vi "运维调试_采配水V2.vi"() -> ()   [LabVIEW 2016, in "PLC.lvlib"]
uses:
  PLC.lvlib
  <vilib>/Plasmionique/MB Master/MB_Master/MB_Master.lvclass
  <vilib>/Utility/miscctls.llb/LVPointTypeDef.ctl
  <vilib>/Plasmionique/MB Master/MB_Master_Serial/MB_Master_Serial.lvclass
  C:/Program Files (x86)/National Instruments/LabVIEW 2016/vi.lib/Plasmionique/MB Master/MB_Master/MB_Master.lvclass
  <vilib>/Instr/_visa.llb/VISA Configure Serial Port (Instr).vi
  <vilib>/NI/Modbus Library/API/Wrapper/Create TCP Slave.vi
  <vilib>/NI/Modbus Library/API/slave/Modbus Slave.lvclass
  <vilib>/Plasmionique/MB Master/MB Master.lvlib
  <vilib>/NI/Modbus Library/API/Wrapper/API Main.lvlib
panel:
  out "Registers":u16[](array[numeric])
  out "R118":i16 caption="多参数沉淀时间"
  in  "看门狗启用":bool
  out "R117":i16 caption="看门狗设置值"
  out "R33":i16 caption="看门狗计时器"
  in  "下载模式":bool
  in  "R116":i16(ring) caption="储水水体选择" items=["自来水", "采水泵"]
  out "当前启动泵号":u16(ring) items=["1号水样泵", "2号水样泵"]
  out "R113":i16 caption="储水时间设定"
  out "R25":i16
  in  "V14NC":bool
  out "R24":i16
  in  "V14NO":bool
  out "X2":bool caption="X1"
  out "采配水版本号":string
  out "R23":i16 caption="清洗频次计数"
  out "R112":i16 caption="清洗频次设定"
  out "R22":i16
  in  "V13NC":bool
  out "R111":i16 caption="排液时间"
  out "通讯故障":bool
  out "R21":i16
  in  "V13NO":bool
  out "R20":i16
  in  "M1-2":bool
  in  "潜水泵工作模式":u16(ring) items=["泵1单泵单管路", "泵2单泵单管路", "潜水泵双泵双管路", "自吸泵双泵双管路"]
  out "X11":bool caption="废液报警"
  out "X10":bool caption="自来水检测"
  out "X9":bool caption="泵2过载报警"
  out "X8":bool caption="泵1过载报警"
  out "X7":bool caption="断电检测"
  out "X6":bool caption="开门检测"
  out "X5":bool caption="烟雾检测"
  out "X4":bool caption="漏水检测"
  out "X3":bool caption="进样检测"
  out "X1":bool
  out "X0":bool caption="采样池液位开关"
  out "R109":i16 caption="配水时间"
  out "集成报警信息":string
  out "R108":i16 caption="自来水报警"
  out "R107":i16 caption="采水池液位报警设置"
  out "R106":i16 caption="进样超时设置"
  out "R105":i16 caption="二级清洗时间"
  out "R104":i16 caption="一级清洗时间"
  out "R103":i16 caption="外部管路清洗时间"
  out "R102":i16 caption="静置沉淀时间"
  out "R101":i16 caption="内部管路润洗时间"
  out "R100":i16 caption="外部管路润洗时间"
  out "R2":i16
  out "R1":i16
  out "多列列表框":i32(listbox)
  out "R19":i16
  in  "V6":bool
  out "R18":i16
  in  "V5":bool
  out "R17":i16
  in  "V4":bool
  out "R16":i16
  in  "V3":bool
  out "R15":i16
  in  "V2":bool
  out "R14":i16
  in  "M2":bool
  out "R13":i16
  in  "V1":bool
  out "R12":i16
  in  "M1-1":bool
  in  "返回":bool
  in  "参数设置":bool
  in  "单步启动":bool
  in  "启动":bool
  in  "停止":bool
  # "看门狗设置"
  # "S"
  # "S"
  # "S"
  # "S"
  # "次"
  # "次"
  # "S"
  # "S"
  # "S"
  # "S"
  # "S"
  # "S"
  # "S"
  # "S"
  # "S"
  # "S"
  # "S"
  # "单步计时："
  # "s"
  # "流程计时："
  # "s"
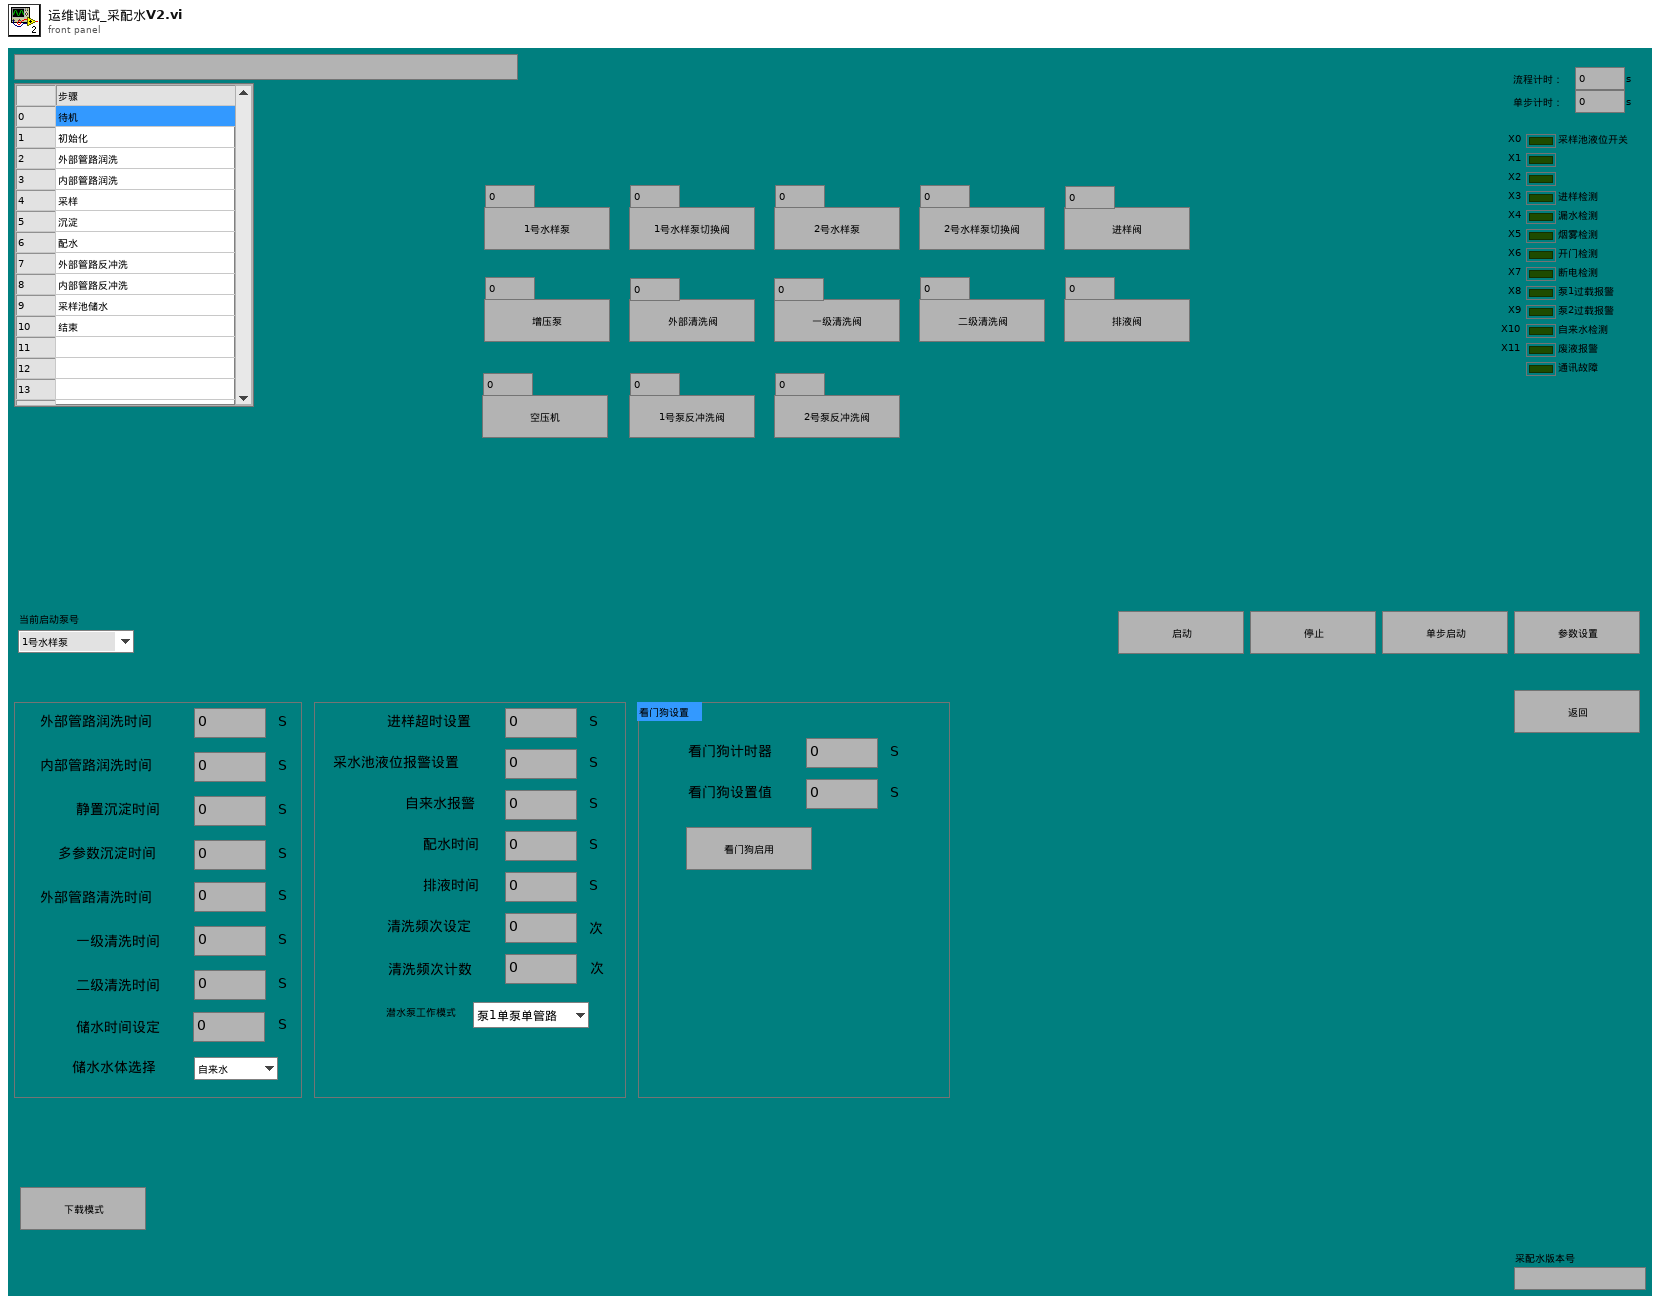
[diagram p1: front panel]
types:
  T1 = typedef "LVPointTypeDef.ctl" = cluster{"Horizontal":i16, "Vertical":i16}
  T2 = cluster{"命令":string, "数据":cluster{"starting address":u16, "holding register value":u16}}
  T3 = cluster{"时间标识":timestamp, "设备":string, "日志信息":string}
  T4 = cluster{"R0":i16, "R1":i16, "R2":i16, "R3":i16, "R4":i16, "R5":i16, "R6":i16, "R7":i16, "R8":i16, "R9":i16, "R10":i16, "R11":i16, "R12":i16, "R13":i16, "R14":i16, "R15":i16, "R16":i16, "R17":i16, "R18":i16, "R19":i16, "R20":i16, "R21":i16, "R22":i16, "R23":i16, "R24":i16, "R25":i16, "R26":i16, "R27":i16, "R28":i16, "R29":i16, "R30":i16, "R31":i16, "R32":i16, "R33":i16, "R34":i16}
  T5 = cluster{"R100":i16, "R101":i16, "R102":i16, "R103":i16, "R104":i16, "R105":i16, "R106":i16, "R107":i16, "R108":i16, "R109":i16, "R110":i16, "R111":i16, "R112":i16, "R113":i16, "R114":i16, "R115":i16, "R116":i16, "R117":i16, "R118":i16, "R119":i16}
  T6 = cluster{"seconds since 1Jan1904":timestamp, "table输入":string, string, "table输入":string}
  T7 = cluster{"时间标识":timestamp, "设备":string, "日志信息":string, "流程参数":string}
  T8 = cluster{"命令":string, cluster{"starting address":u16, "holding register value":u16}}
  T9 = cluster{"命令":string, "数据":cluster{"starting address":u16, "holding register values":u16[]}}
  T10 = cluster{"命令":string, "data":cluster{"starting address":u16, "coil values":bool[]}}
  T11 = cluster{"测试模式":enum16{"正常测试", "集成干预"}, "参数启用":cluster{"氨氮":bool, "总磷总氮":bool, "CODMn":bool, "CODcr":bool, "多参数":bool, "超标留样":bool}}
  T12 = enum32{"Bad", "Idle", "Run top level", "Running"}
  T13 = cluster{"baud rate (bps)":u32, "stop bits":u16, "parity":u16, "flow control":u16, "timeout":u32, "retries":i32}
  T14 = cluster{"starting address":u16, "holding register values":u16[]}
  T15 = cluster{"starting address":u16, "holding register value":u16}
  T16 = cluster{"starting address":u16, "coil values":bool[]}
  T17 = cluster{"Registers[0]":u16, "Registers[1]":u16, "Registers[2]":u16, "Registers[3]":u16, "Registers[4]":u16, "Registers[5]":u16, "Registers[6]":u16, "Registers[7]":u16, "Registers[8]":u16, "Registers[9]":u16, "Registers[10]":u16, "Registers[11]":u16, "Registers[12]":u16, "Registers[13]":u16, "Registers[14]":u16, "Registers[15]":u16, "Registers[16]":u16, "Registers[17]":u16, "Registers[18]":u16, "Registers[19]":u16, "Registers[20]":u16, "Registers[21]":u16, "Registers[22]":u16, "Registers[23]":u16, "Registers[24]":u16, "Registers[25]":u16, "Registers[26]":u16, "Registers[27]":u16, "Registers[28]":u16, "Registers[29]":u16, "Registers[30]":u16, "Registers[31]":u16, "Registers[32]":u16, "Registers[33]":u16, "Registers[34]":u16}
  T18 = cluster{"数组 2[0]":sgl, "数组 2[1]":sgl, "数组 2[2]":sgl, "数组 2[3]":sgl, "数组 2[4]":sgl}
  T19 = cluster{"Registers[0]":u16, "Registers[1]":u16, "Registers[2]":u16, "Registers[3]":u16, "Registers[4]":u16, "Registers[5]":u16}
  T20 = cluster{"Registers[0]":u16, "Registers[1]":u16, "Registers[2]":u16, "Registers[3]":u16, "Registers[4]":u16, "Registers[5]":u16, "Registers[6]":u16, "Registers[7]":u16, "Registers[8]":u16, "Registers[9]":u16, "Registers[10]":u16, "Registers[11]":u16, "Registers[12]":u16, "Registers[13]":u16, "Registers[14]":u16, "Registers[15]":u16, "Registers[16]":u16, "Registers[17]":u16, "Registers[18]":u16, "Registers[19]":u16}
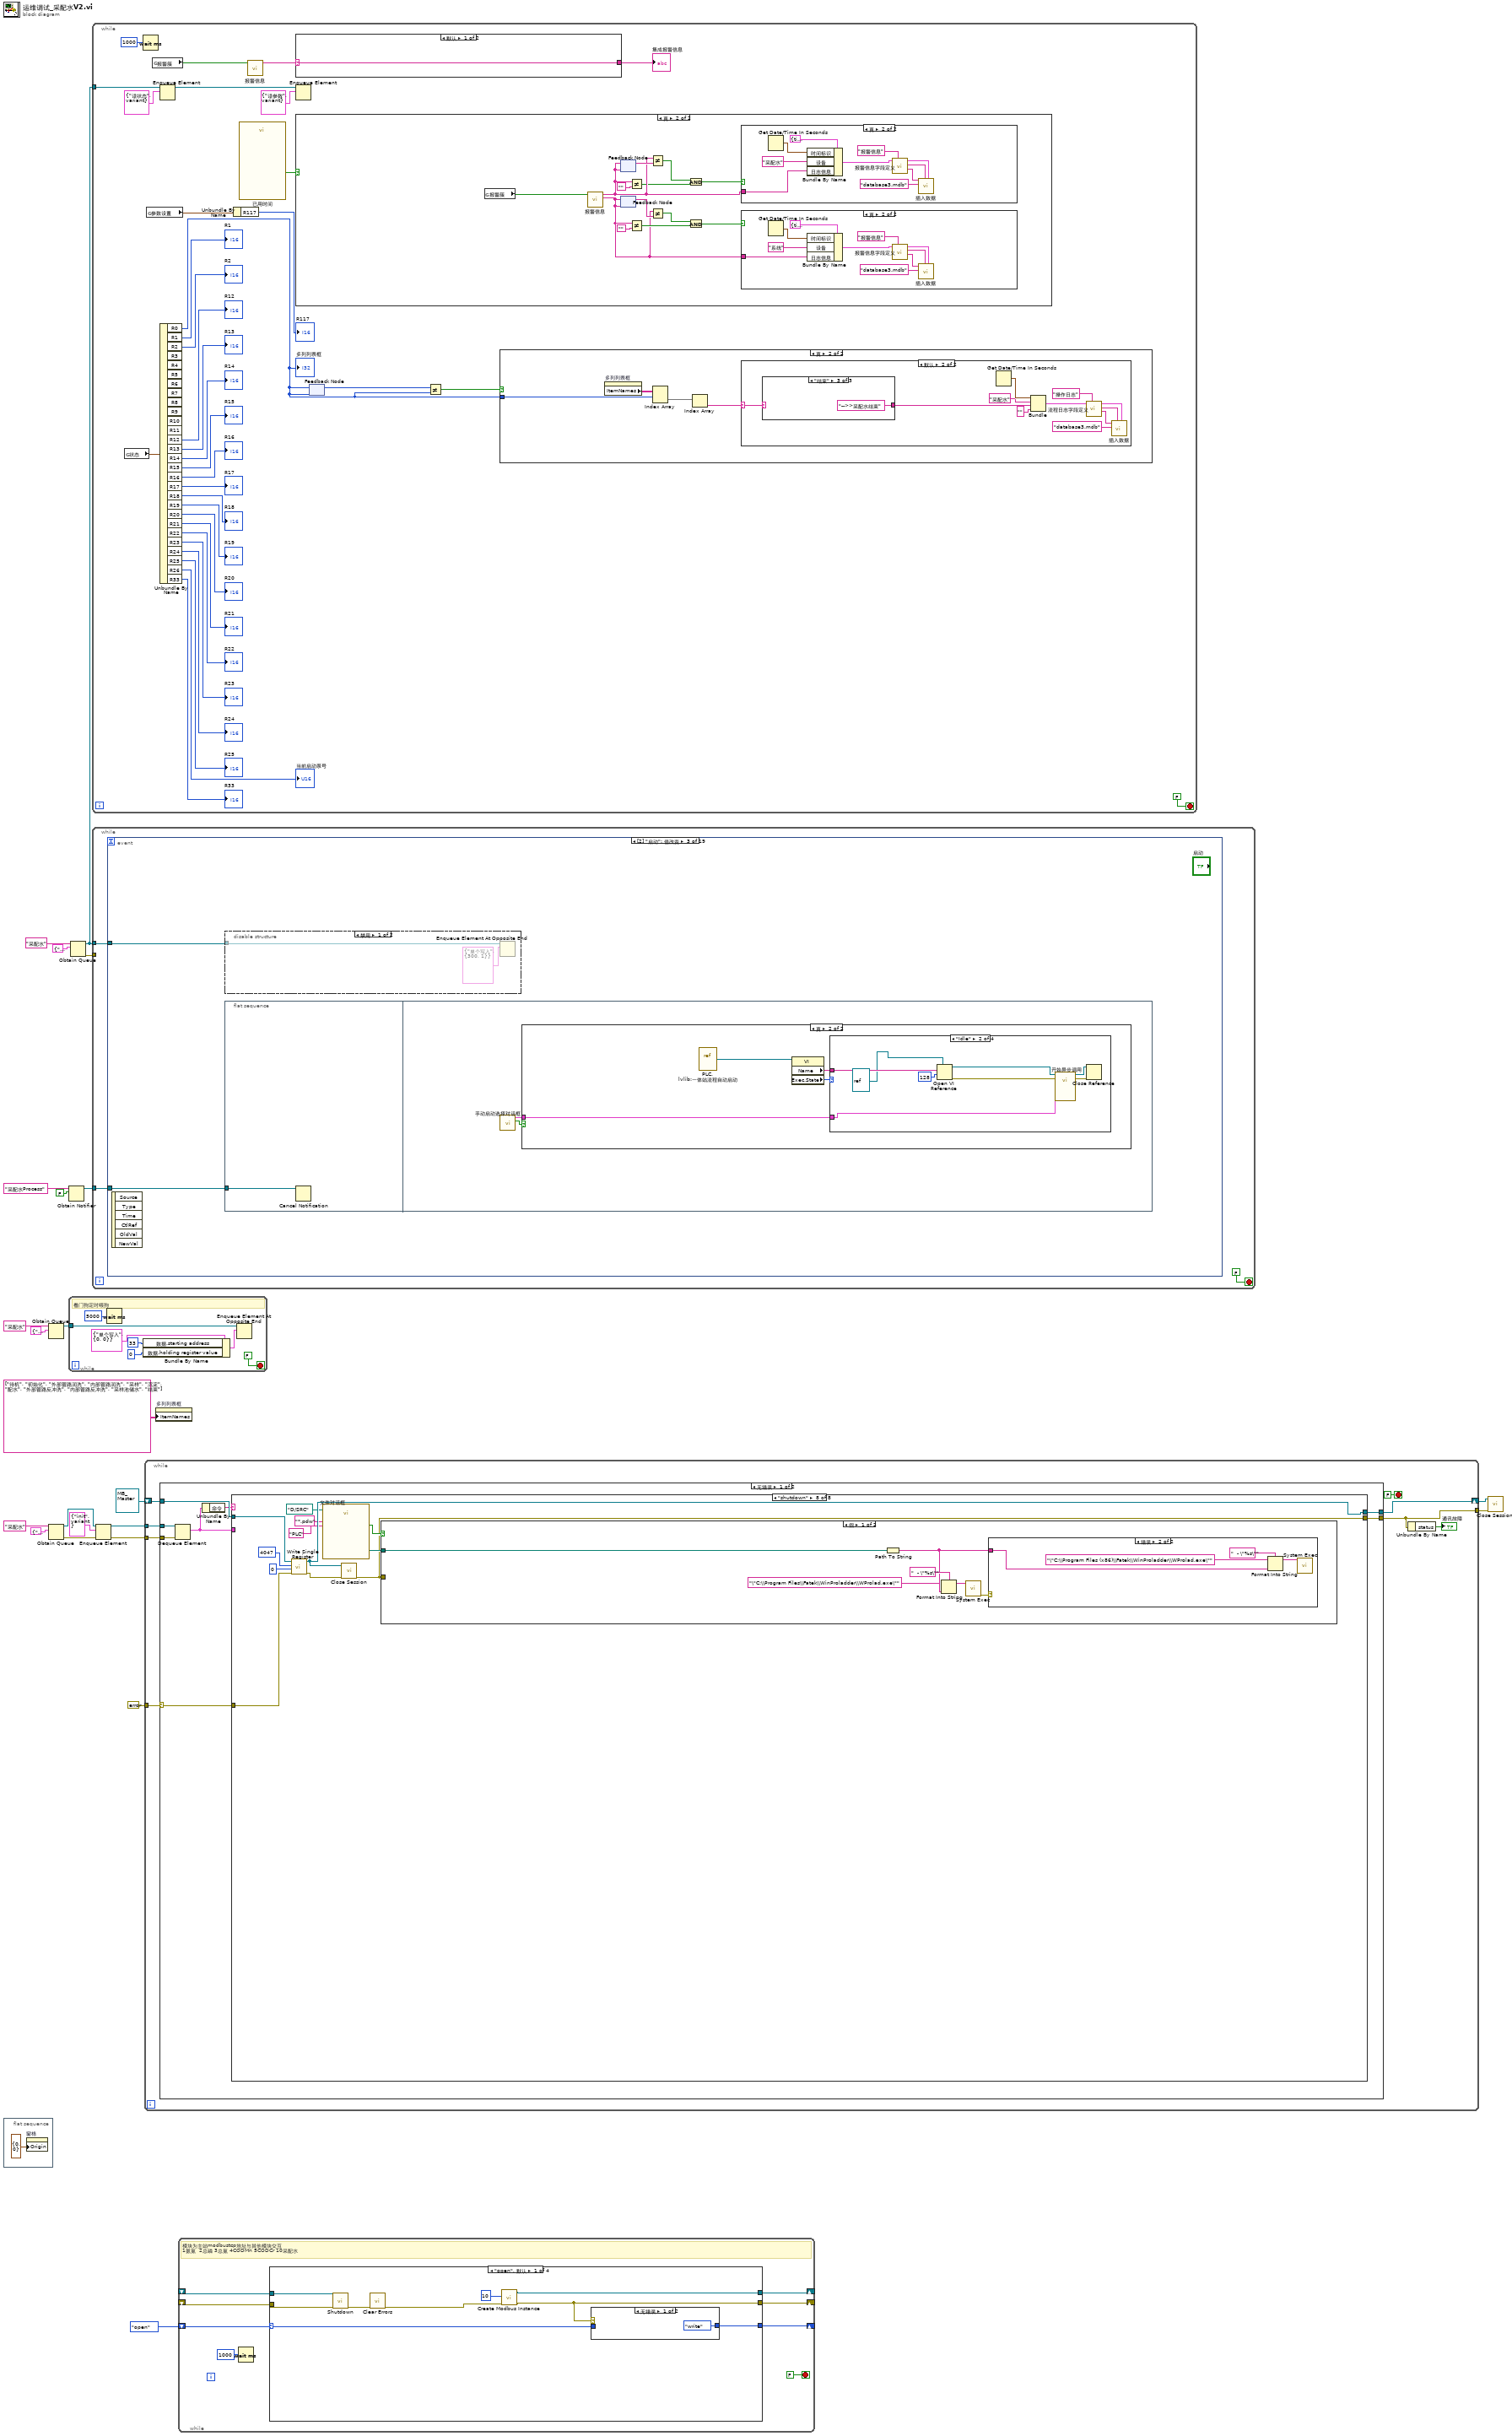
[diagram p0: block diagram]
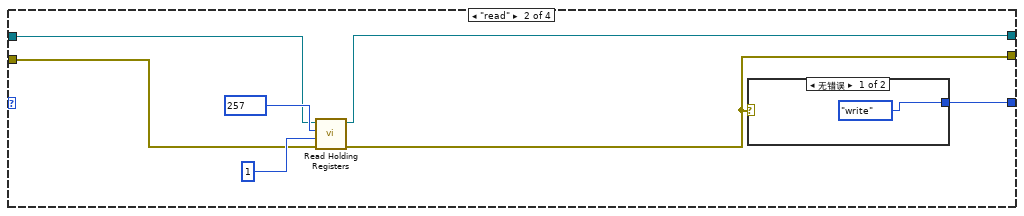
[diagram p3: hidden frame]
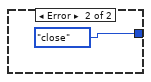
[diagram p4: hidden frame]
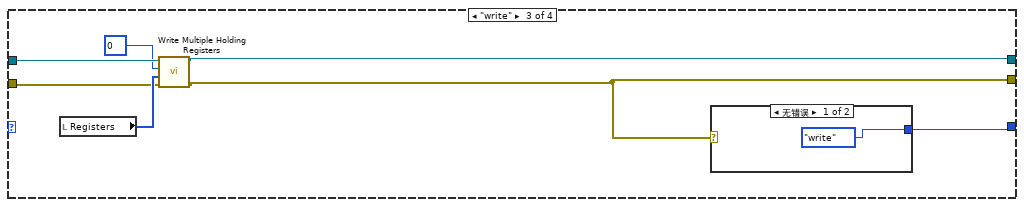
[diagram p5: hidden frame]
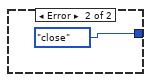
[diagram p6: hidden frame]
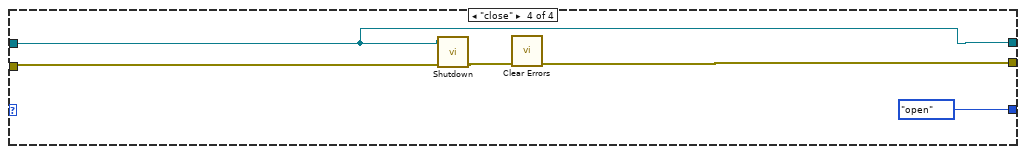
[diagram p7: hidden frame]
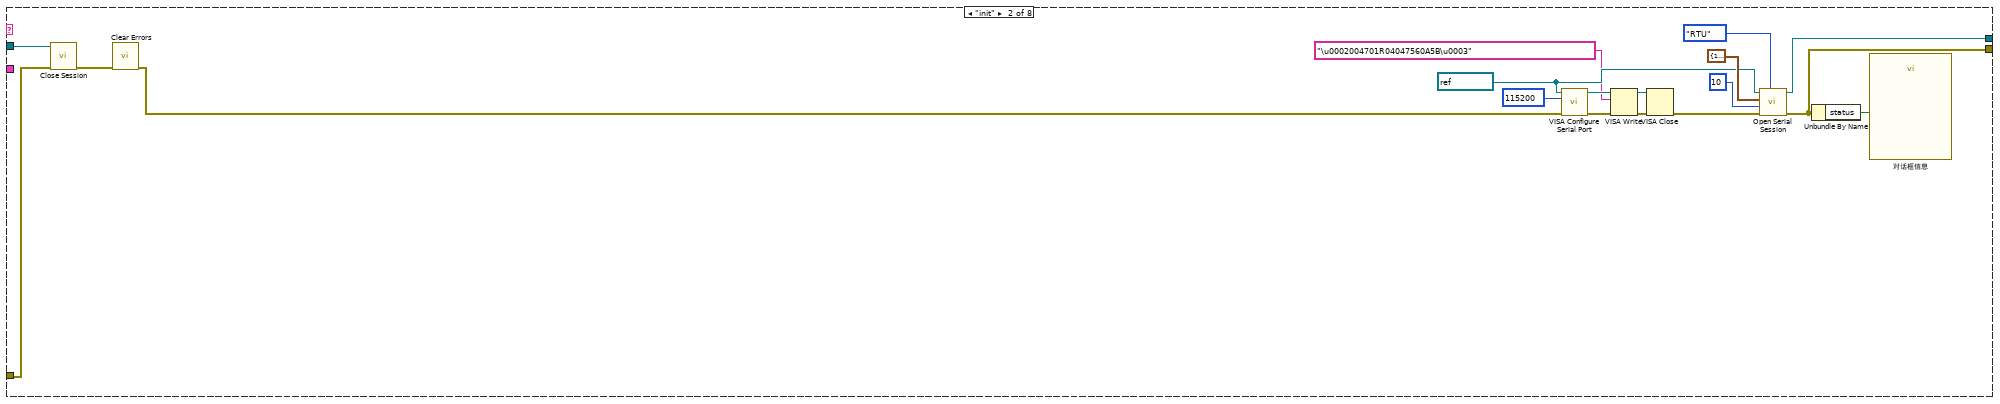
[diagram p9: hidden frame]
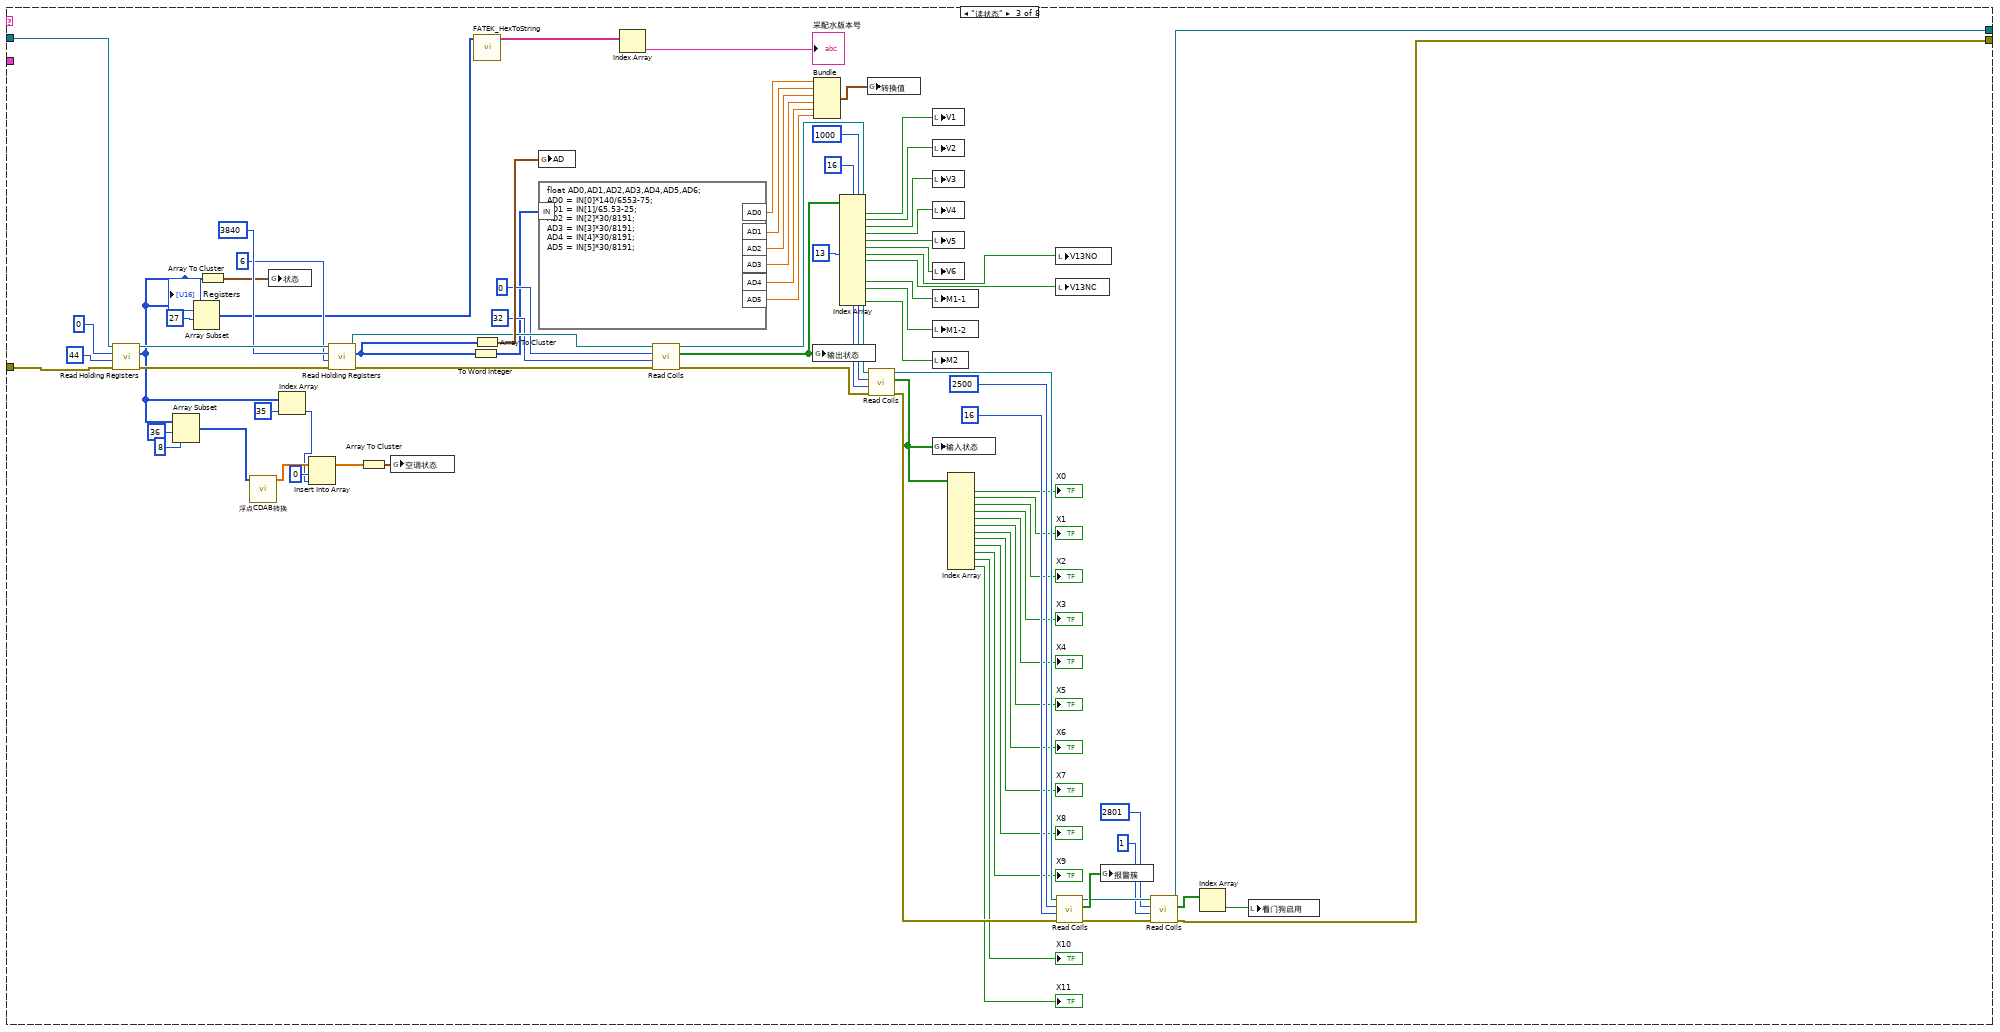
[diagram p10: hidden frame]
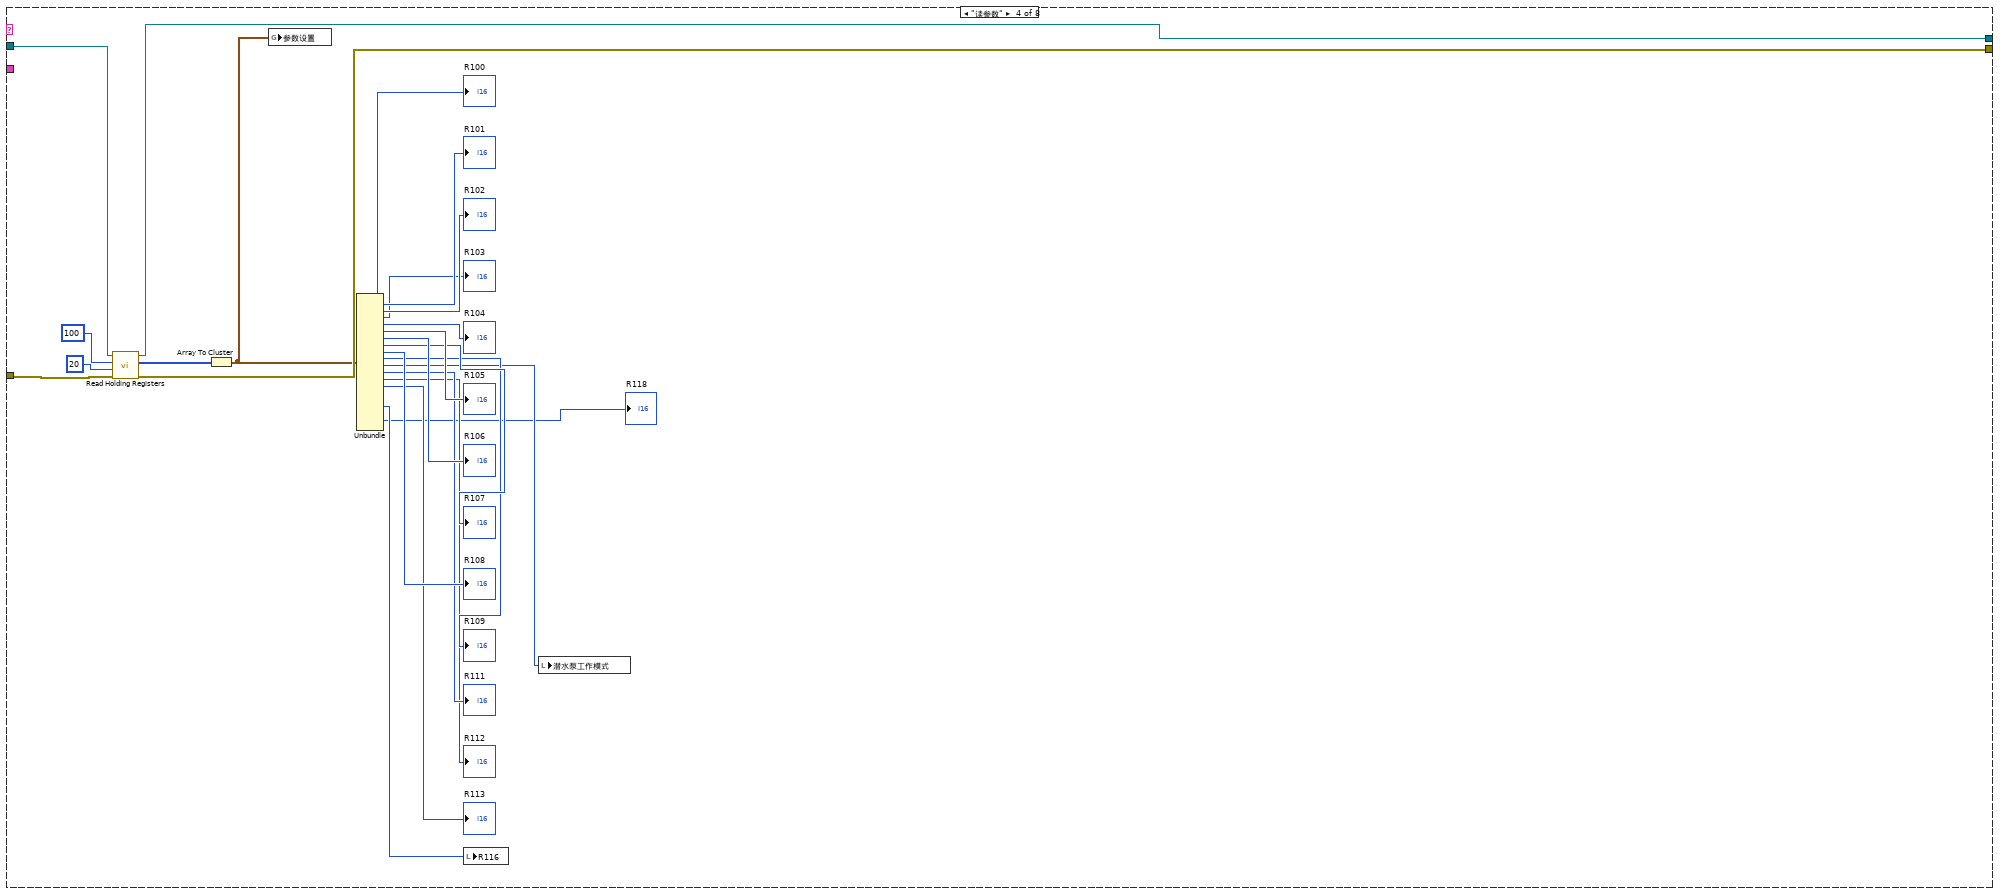
[diagram p11: hidden frame]
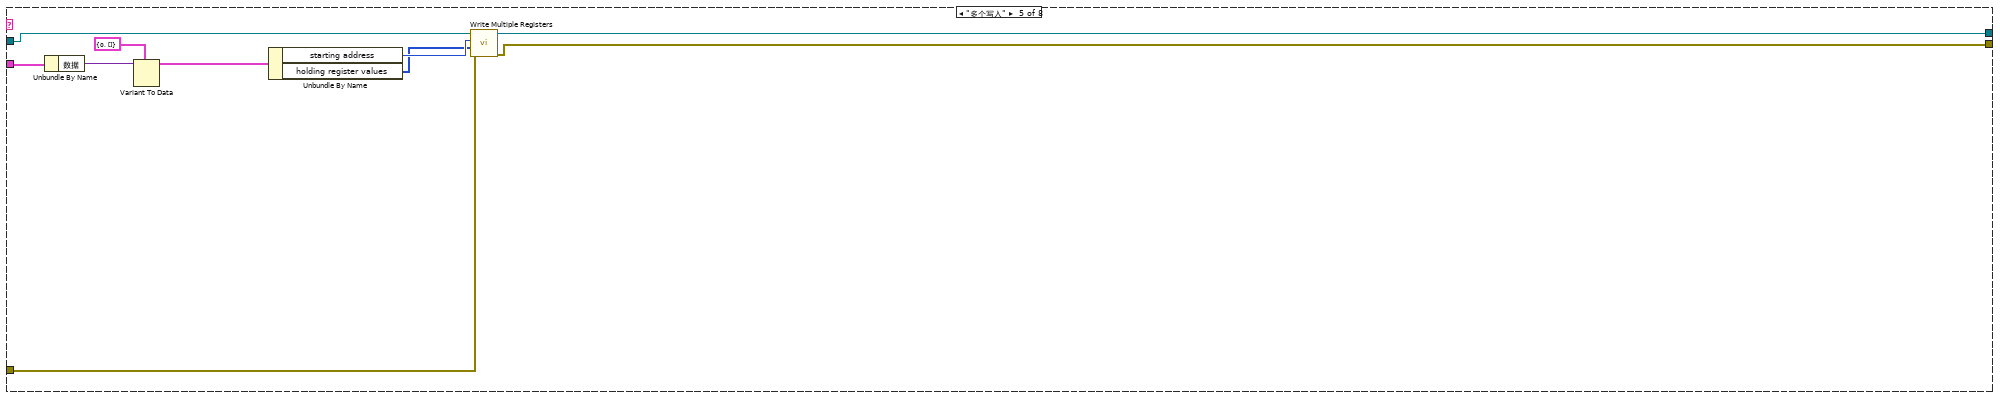
[diagram p12: hidden frame]
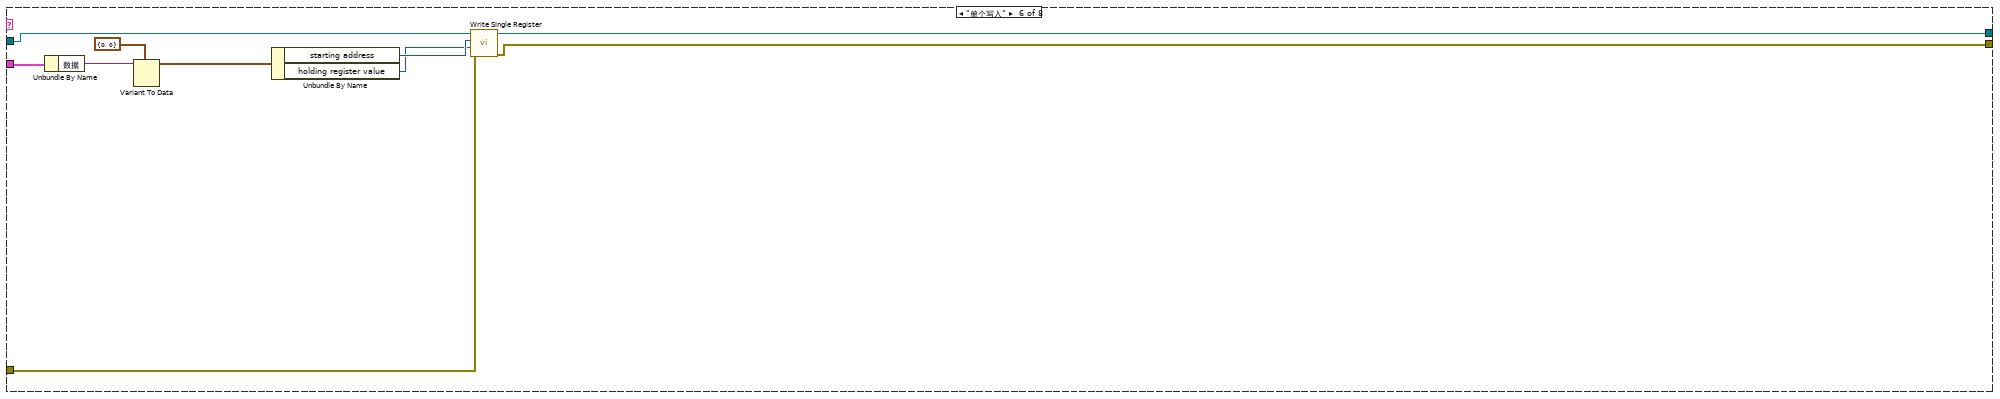
[diagram p13: hidden frame]
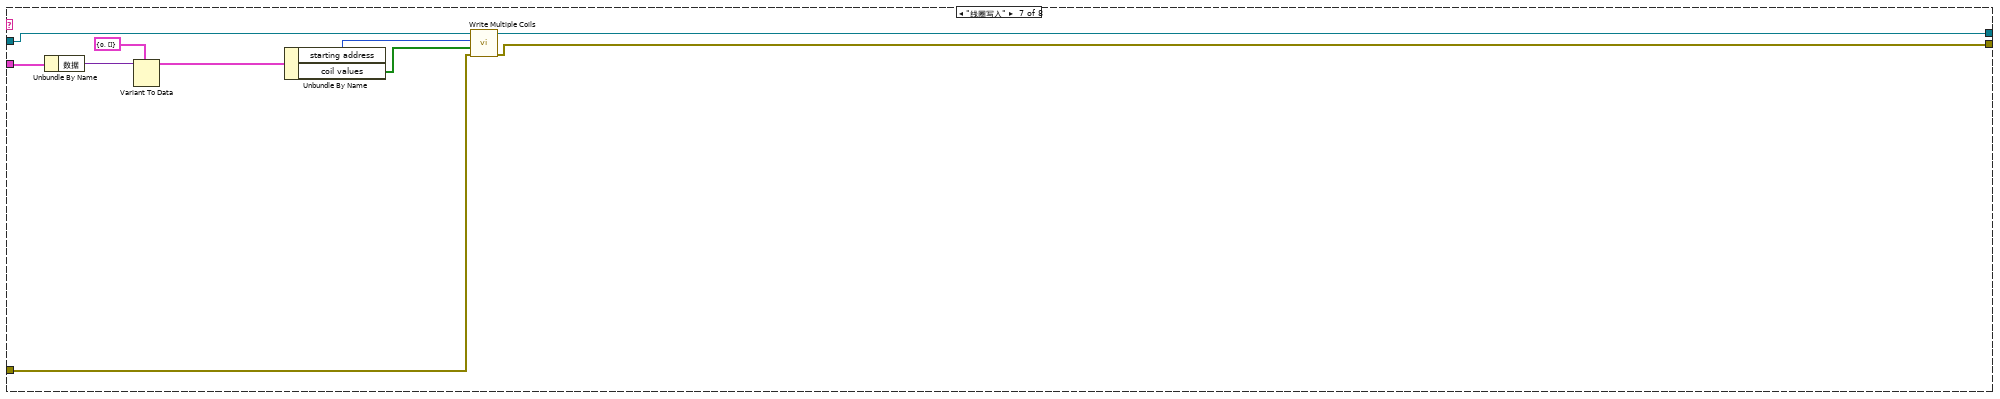
[diagram p14: hidden frame]
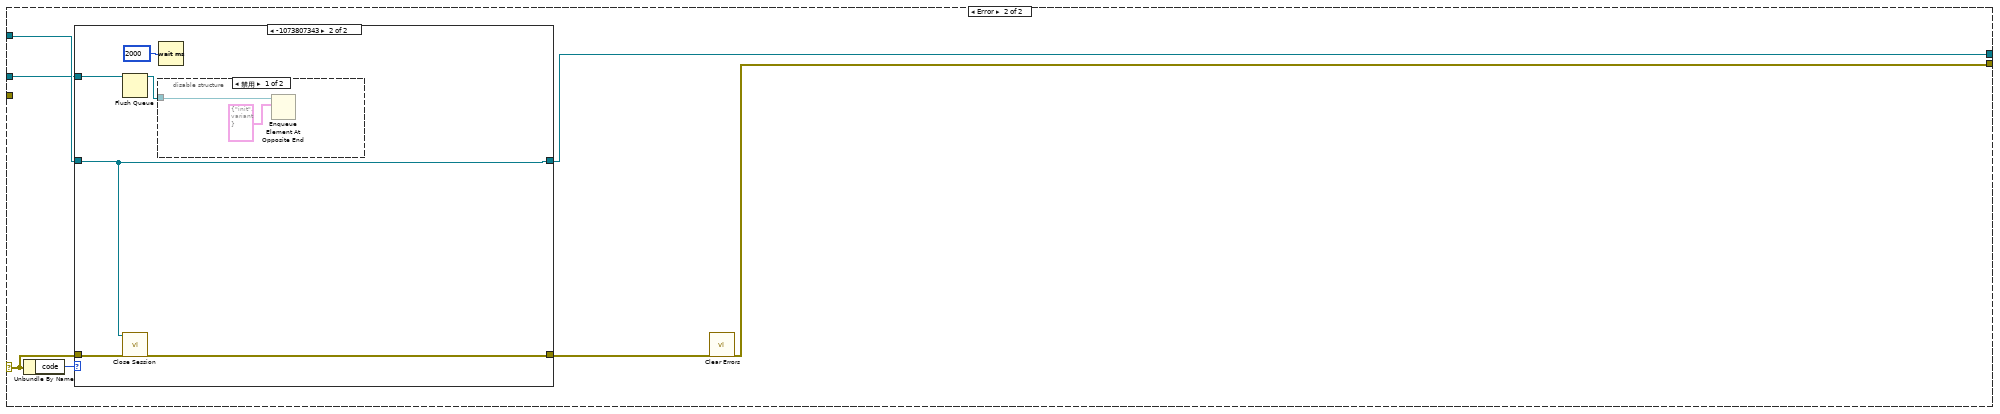
[diagram p17: hidden frame]
diagram:
  n1 = flat-sequence {
    frame #0 {
      n2 = property on="窗格" class="Pane"("Origin"=T1 {"Horizontal"=0, "Vertical"=0} ("原点")) -> ()  [unwired: 2 in, 2 out]
    }
  }
  n3 = Obtain Queue(name (unnamed)="采配水" ("名称（未命名）"), element data type=cluster{"命令":string, "数据":variant} {"命令"="", "数据"=variant}) -> (queue out=w2:refnum<queue>)  [unwired: 3 in, 2 out]
  n4 = Obtain Queue(name (unnamed)="采配水" ("名称（未命名）"), element data type=cluster{"命令":string, "数据":variant} {"命令"="", "数据"=variant}) -> (queue out=w13:refnum<queue>, error out=w12:errorcluster)  [unwired: 3 in, 1 out]
  n5 = Obtain Notifier(name (unnamed)="采配水Process" ("名称（未命名）"), notification data type=FALSE) -> (notifier out=w16:refnum<notifier>)  [unwired: 2 in, 2 out]
  n6 = while {
    tunnel: w2 -> [w27]
    stop <- FALSE stop-if-true
    # "看门狗定时喂狗"
    n7 = Wait (ms)(milliseconds to wait=u32 5000 ("等待时间（毫秒）")) -> ()  [unwired: 1 out]
    n8 = Bundle By Name(cluster=T2 {"命令"="单个写入", "数据"={"starting address"=0, "holding register value"=0}} ("元素"), "数据.starting address"=u16 33, "数据.holding register value"=u16 0) -> (w28:T2)
    n9 = Enqueue Element At Opposite End(queue=w27, element=w28) -> ()  [unwired: 2 in, 3 out]
  }
  n10 = Obtain Queue(name (unnamed)="采配水" ("名称（未命名）"), element data type=cluster{"命令":string, "数据":variant} {"命令"="", "数据"=variant}) -> (queue out=w20:refnum<queue>, error out=w21:errorcluster)  [unwired: 3 in, 1 out]
  n11 = while {
    tunnel: w20 -> [w64]
    stop <- FALSE stop-if-true
    n12 = global read "采配水全局变量.vi" "状态"() -> (w62:T4)
    n13 = Wait (ms)(milliseconds to wait=u32 1000 ("等待时间（毫秒）")) -> ()  [unwired: 1 out]
    n14 = global read "采配水全局变量.vi" "参数设置"() -> (w33:T5)
    n15 = global read "采配水全局变量.vi" "报警簇"() -> (w50:bool[])
    n16 = Enqueue Element(queue=w64, element=cluster{"命令":string, "数据":variant} {"命令"="读状态", "数据"=variant} ("元素")) -> (queue out=w45:refnum<queue>)  [unwired: 2 in, 2 out]
    n17 = Unbundle By Name(w62) -> ("R0"=w43:i16, "R1"=→"R1":i16, "R2"=→"R2":i16, "R12"=→"R12":i16, "R13"=→"R13":i16, "R14"=→"R14":i16, "R15"=→"R15":i16, "R16"=→"R16":i16, "R17"=→"R17":i16, "R18"=→"R18":i16, "R19"=→"R19":i16, "R20"=→"R20":i16, "R21"=→"R21":i16, "R22"=→"R22":i16, "R23"=→"R23":i16, "R24"=→"R24":i16, "R25"=→"R25":i16, "R26"=→"当前启动泵号":i16, "R33"=→"R33":i16)  [unwired: 9 out]
    "多列列表框" <- w43
    n18 = Unbundle By Name(w33) -> ("R117"=→"R117":i16)
    n19 = call "已用时间"() -> ("Time has Elapsed"=w48:bool)  [unwired: 12 in, 7 out]
    n20 = call "报警信息.vi"("报警簇"=w50) -> ("采配水报警信息"=w42:string)  [unwired: 9 in, 1 out]
    n21 = case shown="默认" w42 {
      selector: w42 -> [w99 _]
      tunnel: [w99 w100] -> w49
      frame Default {
      }
      frame "" {
        n22 = global read "采配水全局变量.vi" "运行状态显示"() -> (w100:string)
      }
    }
    "集成报警信息" <- w49
    n23 = Enqueue Element(queue=w45, element=cluster{"命令":string, "数据":variant} {"命令"="读参数", "数据"=variant} ("元素")) -> ()  [unwired: 2 in, 3 out]
    n24 = case shown="真" w48 {
      frame False {
      }
      frame True {
        n25 = global read "采配水全局变量.vi" "报警簇"() -> (w78:bool[])
        n26 = call "报警信息.vi"("报警簇"=w78) -> ("系统报警信息"=w67:string, "采配水报警信息"=w74:string)  [unwired: 9 in]
        n27 = feedback #1(w74) -> (w77:string)
        n28 = feedback-in #1(w74) -> ()
        n29 = feedback #2(w67) -> (w68:string)
        n30 = feedback-in #2(w67) -> ()
        n31 = Not Equal?(x=w74, y="") -> (x != y?=w72:bool)
        n32 = Not Equal?(x=w67, y="") -> (x != y?=w71:bool)
        n33 = Not Equal?(x=w74, y=w77) -> (x != y?=w76:bool)
        n34 = Not Equal?(x=w67, y=w68) -> (x != y?=w69:bool)
        n35 = And(x=w76, y=w72) -> (x .and. y?=w75:bool)
        n36 = And(x=w69, y=w71) -> (x .and. y?=w66:bool)
        n37 = case shown="真" w75 {
          tunnel: w74 -> [_ w89]
          frame False {
          }
          frame True {
            n38 = Get Date/Time In Seconds() -> (seconds since 1Jan1904=w91:timestamp)
            n39 = Bundle By Name(cluster=T3 {"时间标识"=timestamp(0 s since 1904-01-01), "设备"="", "日志信息"=""} ("data in"), "时间标识"=w91, "设备"="采配水", "日志信息"=w89) -> (w92:T3)
            n40 = call "报警信息字段定义.vi"("table输入"="报警信息", "data in"=w92) -> ("table输出"=w96:string, "columns"=w97:string[], "data out"=w98:T3)  [unwired: 7 in]
            n41 = call "插入数据.vi"("data"=w98, "columns"=w97, "database"="database3.mdb", "table"=w96) -> ()  [unwired: 7 in, 1 out]
          }
        }
        n42 = case shown="真" w66 {
          tunnel: w67 -> [_ w79]
          frame False {
          }
          frame True {
            n43 = Get Date/Time In Seconds() -> (seconds since 1Jan1904=w81:timestamp)
            n44 = Bundle By Name(cluster=T3 {"时间标识"=timestamp(0 s since 1904-01-01), "设备"="", "日志信息"=""} ("data in"), "时间标识"=w81, "设备"="系统", "日志信息"=w79) -> (w82:T3)
            n45 = call "报警信息字段定义.vi"("table输入"="报警信息", "data in"=w82) -> ("table输出"=w86:string, "columns"=w87:string[], "data out"=w88:T3)  [unwired: 7 in]
            n46 = call "插入数据.vi"("data"=w88, "columns"=w87, "database"="database3.mdb", "table"=w86) -> ()  [unwired: 7 in, 1 out]
          }
        }
      }
    }
    n47 = feedback-in #3(w43) -> ()
    n48 = feedback #3(w43) -> (w44:i16)
    n49 = Not Equal?(x=w44, y=w43) -> (x != y?=w51:bool)
    n50 = case shown="真" w51 {
      tunnel: w43 -> [_ w103]
      frame False {
      }
      frame True {
        n51 = property on="多列列表框" class="MCListbox (严格)"() -> ("ItemNames"=w104:string[][])  [unwired: 2 in, 2 out]
        n52 = Index Array(array=w104, index (row)=w103) -> (element=w102:string[])  [unwired: 1 in]
        n53 = Index Array(array=w102) -> (element=w101:string)  [unwired: 1 in]
        n54 = case shown="默认" w101 {
          selector: w101 -> [_ w106]
          frame "待机" {
          }
          frame Default {
            n55 = case shown="\"结束\"" w106 {
              selector: w106 -> [w116 _ _]
              tunnel: [w116 "-->>采配水初始化" "-->>采配水结束"] -> w105
              frame Default {
              }
              frame "初始化" {
              }
              frame "结束" {
              }
            }
            n56 = Get Date/Time In Seconds() -> (seconds since 1Jan1904=w110:timestamp)
            n57 = Bundle("seconds since 1Jan1904"=w110, "table输入"="采配水", w105, "table输入"="") -> (w108:T6)  [unwired: 1 in]
            n58 = call "流程日志字段定义.vi"("table输入"="操作日志", "data in"=w108) -> ("table输出"=w113:string, "columns"=w114:string[], "data out"=w115:T7)  [unwired: 7 in]
            n59 = call "插入数据.vi"("data"=w115, "columns"=w114, "database"="database3.mdb", "table"=w113) -> ()  [unwired: 7 in, 1 out]
          }
        }
      }
    }
  }
  n60 = while {
    tunnel: w20 -> [w120]
    tunnel: w21 -> [_]
    tunnel: w16 -> [w119]
    stop <- FALSE stop-if-true
    n61 = event shown="[2] \"启动\": 值改变" {
      selector: _ -> [_ _ _ _ _ _ _ _ _ _ _ _ _ _ _ _ _ _ _]
      dyn-events: _ -> [_ _ _ _ _ _ _ _ _ _ _ _ _ _ _ _ _ _ _]
      timeout: _ -> [_ _ _ _ _ _ _ _ _ _ _ _ _ _ _ _ _ _ _]
      tunnel: w120 -> [_ w124 w127 w149 w168 w173 w179 w190 _ _ _ _ w218 w220 w225 w230 w235 w240 w245]
      tunnel: w119 -> [_ w123 w126 _ _ _ _ _ _ _ _ _ _ _ _ _ _ _ _]
      event Timeout {
        n62 = event-data() -> ()  [unwired: 1 in, 3 out]
      }
      event "停止": Value Change {
        n63 = event-data() -> ()  [unwired: 1 in, 6 out]
        n64 = Send Notification(notification=TRUE ("通知"), notifier=w123) -> ()  [unwired: 1 in, 2 out]
        n65 = Enqueue Element At Opposite End(queue=w124, element=T8 {"命令"="单个写入", {"starting address"=300, "holding register value"=2}} ("元素")) -> ()  [unwired: 2 in, 3 out]
      }
      event "启动": Value Change {
        n66 = event-data() -> ()  [unwired: 1 in, 6 out]
        n67 = disable-structure shown="禁用" {
          disable-tunnel: w127 -> [w145 _]
          frame Disabled {
            n68 = Enqueue Element At Opposite End(queue=w145, element=T8 {"命令"="单个写入", {"starting address"=300, "holding register value"=1}} ("元素")) -> ()  [unwired: 2 in, 3 out]
          }
          frame Enabled {
          }
        }
        n69 = flat-sequence {
          tunnel: w126 -> [w128]
          frame #0 {
            n70 = Cancel Notification(0:w128) -> ()  [unwired: 1 in, 3 out]
          }
          frame #1 {
            n71 = call "手动启动选择对话框.vi"() -> ("确定"=w130:bool, "参数"=w129:T11)  [unwired: 10 in]
            n72 = case shown="真" w130 {
              tunnel: w129 -> [_ w131]
              frame False {
              }
              frame True {
                n73 = vi-ref "PLC.lvlib:一体站流程自动启动.vi"() -> (w134:refnum<vi>)
                n74 = property class="VI"(reference=w134) -> ("Name"=w133:string, "Exec.State"=w132:T12)  [unwired: 1 in, 2 out]
                n75 = case shown="\"Idle\"" w132 {
                  tunnel: w133 -> [_ w142 _ _]
                  tunnel: w131 -> [_ w136 _ _]
                  frame "Bad", Default {
                  }
                  frame "Idle" {
                    n76 = Open VI Reference(type specifier VI Refnum (for type only)=refnum<vi> refnum, vi path=w142, options=128 ("选项")) -> (vi reference=w140:refnum<vi>, error out=w138:errorcluster)  [unwired: 3 in]
                    n77 = call-by-ref "开始异步调用"(reference=w140, error in=w138, "参数"=w136) -> (reference out=w139:refnum<vi>, error out=w137:errorcluster)  [unwired: 11 in]
                    n78 = Close Reference(reference=w139, error in (no error)=w137) -> ()  [unwired: 1 out]
                  }
                  frame "Run top level" {
                  }
                  frame "Running" {
                    n79 = One Button Dialog(message="流程已经运行,无须重复启动" ("消息")) -> ()  [unwired: 1 in, 1 out]
                  }
                }
              }
            }
          }
        }
      }
      event "单步启动": Value Change {
        n80 = event-data() -> ()  [unwired: 1 in, 6 out]
        n81 = call "单步启动对话框.vi"() -> ("单步启动步骤输出"=w146:u16)  [unwired: 11 in]
        n82 = Bundle By Name(cluster=T2 {"命令"="单个写入", "数据"={"starting address"=301, "holding register value"=0}} ("元素"), "数据.holding register value"=w146) -> (w147:T2)
        n83 = Enqueue Element At Opposite End(queue=w149, element=w147) -> ()  [unwired: 2 in, 3 out]
      }
      event "R100", "R101", "R102", "R103", "R104", "R105", "R106", "R107", "R108", "R109", "潜水泵工作模式", "R111", "R112", "R113": Value Change {
        n84 = event-data() -> ()  [unwired: 1 in, 6 out]
        n85 = local read "R100"() -> (w163:i16)
        n86 = local read "R101"() -> (w162:i16)
        n87 = local read "R102"() -> (w161:i16)
        n88 = local read "R103"() -> (w160:i16)
        n89 = local read "R104"() -> (w159:i16)
        n90 = local read "R105"() -> (w158:i16)
        n91 = local read "R106"() -> (w157:i16)
        n92 = local read "R107"() -> (w156:i16)
        n93 = local read "R108"() -> (w155:i16)
        n94 = local read "R109"() -> (w154:i16)
        n95 = local read "R111"() -> (w152:i16)
        n96 = local read "R112"() -> (w151:i16)
        n97 = local read "R113"() -> (w150:i16)
        n98 = Build Array(w163, w162, w161, w160, w159, w158, w157, w156, w155, w154, "潜水泵工作模式", w152, w151, w150) -> (w164:u16[])
        n99 = Bundle By Name(cluster=T9 {"命令"="多个写入", "数据"={"starting address"=0, "holding register values"=[]}} ("元素"), "数据.starting address"=u16 100, "数据.holding register values"=w164) -> (w165:T9)
        n100 = Enqueue Element At Opposite End(queue=w168, element=w165) -> ()  [unwired: 2 in, 3 out]
      }
      event "R116", "R117", "R118": Value Change {
        n101 = event-data() -> ()  [unwired: 1 in, 6 out]
        n102 = local read "R117"() -> (w170:i16)
        n103 = local read "R118"() -> (w169:i16)
        n104 = Build Array("R116", w170, w169) -> (w172:i16[])
        n105 = Bundle By Name(cluster=T9 {"命令"="多个写入", "数据"={"starting address"=0, "holding register values"=[]}} ("元素"), "数据.starting address"=u16 116, "数据.holding register values"=w172) -> (w174:T9)
        n106 = Enqueue Element At Opposite End(queue=w173, element=w174) -> ()  [unwired: 2 in, 3 out]
      }
      event "下载模式": Value Change {
        n107 = event-data() -> ("NewVal"=w178:bool)  [unwired: 1 in, 5 out]
        n108 = Flush Queue(queue=w179) -> (queue out=w177:refnum<queue>)  [unwired: 1 in, 2 out]
        n109 = case shown="真" w178 {
          tunnel: w177 -> [w180 w184]
          frame False {
            n110 = Enqueue Element At Opposite End(queue=w180, element=cluster{"命令":string, "数据":variant} {"命令"="init", "数据"=variant} ("元素")) -> ()  [unwired: 2 in, 3 out]
          }
          frame True {
            n111 = Two Button Dialog(message="请再次确认是否切换为下载模式，切换为下载模式将导致采配水工作异常，非专业人员请勿进行此操作！" ("消息")) -> (T button?=w182:bool)  [unwired: 2 in]
            n112 = case shown="真" w182 {
              tunnel: w184 -> [_ w187]
              frame False {
                n113 = local write "下载模式"(FALSE ("下载模式")) -> ()
              }
              frame True {
                n114 = Enqueue Element At Opposite End(queue=w187, element=cluster{"命令":string, "数据":variant} {"命令"="shutdown", "数据"=variant} ("元素")) -> ()  [unwired: 2 in, 3 out]
              }
            }
          }
        }
      }
      event "R23": Value Change {
        n115 = event-data() -> ()  [unwired: 1 in, 6 out]
        n116 = local read "R23"() -> (w189:i16)
        n117 = Build Array(w189) -> (w188:i16[])
        n118 = Bundle By Name(cluster=T9 {"命令"="多个写入", "数据"={"starting address"=0, "holding register values"=[]}} ("元素"), "数据.starting address"=u16 23, "数据.holding register values"=w188) -> (w191:T9)
        n119 = Enqueue Element At Opposite End(queue=w190, element=w191) -> ()  [unwired: 2 in, 3 out]
      }
      event "R23": Mouse Down {
        n120 = event-data() -> ("CtlRef"=w196:refnum<vi>)  [unwired: 1 in, 7 out]
        n121 = Two Button Dialog(message="请确认是否更改，更改后将影响实际清洗频次" ("消息")) -> (T button?=w195:bool)  [unwired: 2 in]
        n122 = case shown="真" w195 {
          tunnel: w196 -> [_ w197]
          frame False {
          }
          frame True {
            n123 = property class="DigNum (严格)"(reference=w197) -> (reference out=w199:refnum<vi>, "Value"=w200:i16)  [unwired: 1 in, 1 out]
            n124 = call "数字键盘.vi"("OldNumber"=w200) -> ("NewNumber"=w198:sgl)
            n125 = property class="DigNum (严格)"(reference=w199, "Val(Sgnl)"=w198) -> ()  [unwired: 1 in, 2 out]
          }
        }
      }
      event "R100", "R101", "R102", "R103", "R104", "R105", "R106", "R107", "R108", "R109", "R111", "R112", "R113", "R117", "R118": Mouse Down {
        n126 = event-data() -> ("CtlRef"=w204:refnum<vi>)  [unwired: 1 in, 7 out]
        n127 = property class="DigNum (严格)"(reference=w204) -> (reference out=w202:refnum<vi>, "Value"=w203:i16)  [unwired: 1 in, 1 out]
        n128 = call "数字键盘.vi"("OldNumber"=w203) -> ("NewNumber"=w201:sgl)
        n129 = property class="DigNum (严格)"(reference=w202, "Val(Sgnl)"=w201) -> ()  [unwired: 1 in, 2 out]
      }
      event "参数设置": Value Change {
        n130 = event-data() -> ()  [unwired: 1 in, 6 out]
        n131 = property on="窗格" class="Pane"("Origin"=T1 {"Horizontal"=0, "Vertical"=628} ("原点")) -> ()  [unwired: 2 in, 2 out]
      }
      event "返回": Value Change {
        n132 = event-data() -> ()  [unwired: 1 in, 6 out]
        n133 = property on="窗格" class="Pane"("Origin"=T1 {"Horizontal"=0, "Vertical"=0} ("原点")) -> ()  [unwired: 2 in, 2 out]
      }
      event "M1-1", "V1", "M2", "V2", "V3", "V4", "V5", "V6": Value Change {
        n134 = event-data() -> ()  [unwired: 1 in, 6 out]
        n135 = Build Array("M1-1", "V1", "M2", "V2", "V3", "V4", "V5", "V6") -> (w207:bool[])
        n136 = Bundle By Name(cluster=T10 {"命令"="线圈写入", "data"={"starting address"=2400, "coil values"=[]}} ("元素"), "data.coil values"=w207) -> (w208:T10)
        n137 = Enqueue Element(queue=w218, element=w208) -> ()  [unwired: 2 in, 3 out]
      }
      event "M1-2": Value Change {
        n138 = event-data() -> ()  [unwired: 1 in, 6 out]
        n139 = Build Array("M1-2") -> (w221:bool[])
        n140 = Bundle By Name(cluster=T10 {"命令"="线圈写入", "data"={"starting address"=2413, "coil values"=[]}} ("元素"), "data.coil values"=w221) -> (w222:T10)
        n141 = Enqueue Element(queue=w220, element=w222) -> ()  [unwired: 2 in, 3 out]
      }
      event "看门狗启用": Value Change {
        n142 = event-data() -> ()  [unwired: 1 in, 6 out]
        n143 = Build Array("看门狗启用") -> (w226:bool[])
        n144 = Bundle By Name(cluster=T10 {"命令"="线圈写入", "data"={"starting address"=2801, "coil values"=[]}} ("元素"), "data.coil values"=w226) -> (w227:T10)
        n145 = Enqueue Element(queue=w225, element=w227) -> ()  [unwired: 2 in, 3 out]
      }
      event "V13NO": Value Change {
        n146 = event-data() -> ()  [unwired: 1 in, 6 out]
        n147 = Build Array("V13NO") -> (w231:bool[])
        n148 = Bundle By Name(cluster=T10 {"命令"="线圈写入", "data"={"starting address"=2414, "coil values"=[]}} ("元素"), "data.coil values"=w231) -> (w232:T10)
        n149 = Enqueue Element(queue=w230, element=w232) -> ()  [unwired: 2 in, 3 out]
      }
      event "V13NC": Value Change {
        n150 = event-data() -> ()  [unwired: 1 in, 6 out]
        n151 = Build Array("V13NC") -> (w236:bool[])
        n152 = Bundle By Name(cluster=T10 {"命令"="线圈写入", "data"={"starting address"=2415, "coil values"=[]}} ("元素"), "data.coil values"=w236) -> (w237:T10)
        n153 = Enqueue Element(queue=w235, element=w237) -> ()  [unwired: 2 in, 3 out]
      }
      event "V14NO": Value Change {
        n154 = event-data() -> ()  [unwired: 1 in, 6 out]
        n155 = Build Array("V14NO") -> (w241:bool[])
        n156 = Bundle By Name(cluster=T10 {"命令"="线圈写入", "data"={"starting address"=2408, "coil values"=[]}} ("元素"), "data.coil values"=w241) -> (w242:T10)
        n157 = Enqueue Element(queue=w240, element=w242) -> ()  [unwired: 2 in, 3 out]
      }
      event "V14NC": Value Change {
        n158 = event-data() -> ()  [unwired: 1 in, 6 out]
        n159 = Build Array("V14NC") -> (w246:bool[])
        n160 = Bundle By Name(cluster=T10 {"命令"="线圈写入", "data"={"starting address"=2409, "coil values"=[]}} ("元素"), "data.coil values"=w246) -> (w247:T10)
        n161 = Enqueue Element(queue=w245, element=w247) -> ()  [unwired: 2 in, 3 out]
      }
    }
  }
  n162 = Enqueue Element(queue=w13, element=cluster{"命令":string, "数据":variant} {"命令"="init", "数据"=variant} ("元素"), error in (no error)=w12) -> (queue out=w8:refnum<queue>, error out=w10:errorcluster)  [unwired: 1 in, 1 out]
  n163 = while {
    tunnel: w8 -> [w253]
    tunnel: w10 -> [w252]
    shift-right: [w256] -> w5
    shift-left: refnum<class "MB_Master.lvclass"> refnum ("MB session in") -> [w255]
    tunnel: errorcluster {"status"=FALSE, "code"=0, "source"=""} ("error out") -> [w254]
    tunnel: [w251] -> w6
    stop <- FALSE stop-if-true
    n164 = case shown="无错误" w254 {
      selector: w254 -> [w261 w445]
      tunnel: [w264 w444] -> w256
      tunnel: w255 -> [w263 w446]
      tunnel: [w262 w442] -> w251
      tunnel: w253 -> [w259 w441]
      tunnel: w252 -> [w258 _]
      frame No Error {
        n165 = Dequeue Element(queue=w259, error in (no error)=w258) -> (element=w257:cluster{"命令":string, "数据":variant})  [unwired: 1 in, 3 out]
        n166 = Unbundle By Name(w257) -> ("命令"=w260:string)
        n167 = case shown="\"shutdown\"" w260 {
          tunnel: [w266 w279 w302 w383 w395 w405 w415 w427] -> w264
          tunnel: w263 -> [w266 w281 w353 w388 w398 w408 w418 w430]
          tunnel: [w265 w280 w300 w382 w396 w406 w416 w421] -> w262
          tunnel: w261 -> [w265 w283 w356 w387 w397 w407 w417 w428]
          tunnel: w257 -> [_ _ _ _ w394 w404 w414 _]
          frame "idle", Default {
          }
          frame "init" {
            w271 = refnum<visa-resource-name> "COM3" ("VISA resource name")
            n168 = call-dynamic "Close Session.vi"("error in (no error)"=w283, "MB session in"=w281) -> ("error out"=w282:errorcluster)  [unwired: 9 in]
            n169 = call <vilib>:"Clear Errors.vi"("error in (no error)"=w282) -> ("error out"=w269:errorcluster)  [unwired: 5 in, 1 out]
            n170 = call-poly "VISA Configure Serial Port"("VISA resource name"=w271, "baud rate (9600)"=u32 115200, "error in (no error)"=w269) -> ("VISA resource name out"=w273:refnum<visa-resource-name>, "error out"=w275:errorcluster)  [unwired: 11 in]
            n171 = VISA Write(VISA resource name=w273, write buffer="\u0002004701R04047560A5B\u0003" ("写入缓冲区"), error in (no error)=w275) -> (VISA resource name out=w272:refnum<visa-resource-name>, error out=w274:errorcluster)  [unwired: 1 out]
            n172 = VISA Close(VISA resource name=w272, error in (no error)=w274) -> (error out=w268:errorcluster)
            n173 = call <vilib>:"Open Serial Session.vi"("Mode (RTU)"=enum16{"RTU", "ASCII"}."RTU", "Error in"=w268, "Slave ID"=u8 10, "Serial Config"=T13 {"baud rate (bps)"=115200, "stop bits"=10, "parity"=0, "flow control"=0, "timeout"=500, "retries"=1}, "VISA Resource"=w271) -> ("Error out"=w280:errorcluster, "MB_Serial session"=w279:refnum<class "MB_Master_Serial.lvclass">)  [unwired: 5 in]
            n174 = Unbundle By Name(w280) -> ("status"=w284:bool)
            n175 = call "对话框信息"("Enable"=w284) -> ()  [unwired: 9 in, 2 out]
          }
          frame "读状态" {
            n176 = call <vilib>:"Read Holding Registers.vi"("error in (no error)"=w356, "quantity"=u16 44 ("number of holding registers"), "starting address"=u16 0, "MB session in"=w353) -> ("error out"=w351:errorcluster, "Registers"=w289:u16[], "MB session out"=w352:refnum<class "MB_Master.lvclass">)  [unwired: 5 in]
            "Registers" <- w289
            n177 = Array Subset(array=w289, index=36 ("索引"), length=8 ("长度")) -> (w292:u16[])
            n178 = Array Subset(array=w289, index=27 ("索引")) -> (w321:u16[])  [unwired: 1 in]
            n179 = Array To Cluster(array=w289) -> (cluster=w295:T17)
            n180 = call "浮点CDAB转换.vi"("数组"=w292) -> ("数组 2"=w291:sgl[])  [unwired: 10 in]
            n181 = global write "采配水全局变量.vi" "状态"(w295) -> ()
            n182 = Index Array(array=w289, index=35 ("索引")) -> (element=w287:u16)
            n183 = Insert Into Array(array=w291, index=0 ("索引"), new element=w287) -> (w286:sgl[])
            n184 = call <vilib>:"Read Holding Registers.vi"("error in (no error)"=w351, "quantity"=u16 6 ("number of holding registers"), "starting address"=u16 3840, "MB session in"=w352) -> ("error out"=w347:errorcluster, "Registers"=w324:u16[], "MB session out"=w348:refnum<class "MB_Master.lvclass">)  [unwired: 5 in]
            n185 = Array To Cluster(array=w286) -> (cluster=w285:T18)
            n186 = global write "采配水全局变量.vi" "空调状态"(w285) -> ()
            n187 = To Word Integer(number=w324) -> (16bit integer=w323:i16[])
            n188 = call "FATEK_HexToString.vi"("数组"=w321) -> ("STRING"=w320:string[])  [unwired: 10 in]
            n189 = Array To Cluster(array=w324) -> (cluster=w364:T19)
            n190 = global write "采配水全局变量.vi" "AD"(w364) -> ()
            n191 = formula code="float AD0,AD1,AD2,AD3,AD4,AD5,AD6;\nAD0 = IN[0]*140/6553-75;\nAD1 = IN[1]/65.53-25;\nAD2 = IN[2]*30/8191;\nAD3 = IN[3]*30/8191;\nAD4 = IN[4]*30/8191;\nAD5 = IN[5]*30/8191;"("IN"=w323) -> ("AD0"=w362:dbl, "AD1"=w361:dbl, "AD2"=w360:dbl, "AD3"=w359:dbl, "AD4"=w358:dbl, "AD5"=w357:dbl)
            n192 = Index Array(array=w320) -> (element=→"采配水版本号":string)  [unwired: 1 in]
            n193 = call <vilib>:"Read Coils.vi"("error in (no error)"=w347, "quantity"=u16 32 ("number of coils"), "starting address"=u16 0, "MB session in"=w348) -> ("error out"=w343:errorcluster, "Coils"=w328:bool[], "MB session out"=w344:refnum<class "MB_Master.lvclass">)  [unwired: 5 in]
            n194 = global write "采配水全局变量.vi" "输出状态"(w328) -> ()
            n195 = Bundle(w362, w361, w360, w359, w358, w357) -> (w363:cluster{dbl, dbl, dbl, dbl, dbl, dbl})  [unwired: 1 in]
            n196 = Index Array(array=w328, index #7=13 ("索引")) -> (element #1=w318:bool, element #2=w317:bool, element #3=w316:bool, element #4=w315:bool, element #5=w314:bool, element #6=w313:bool, element #7=w311:bool, element #8=w310:bool, element #11=w309:bool, element #12=w308:bool, element #14=w304:bool)  [unwired: 13 in, 3 out]
            n197 = global write "采配水全局变量.vi" "转换值"(w363) -> ()
            n198 = call <vilib>:"Read Coils.vi"("error in (no error)"=w343, "quantity"=u16 16 ("number of coils"), "starting address"=u16 1000, "MB session in"=w344) -> ("error out"=w339:errorcluster, "Coils"=w335:bool[], "MB session out"=w340:refnum<class "MB_Master.lvclass">)  [unwired: 5 in]
            n199 = local write "V1"(w318) -> ()
            n200 = local write "V2"(w317) -> ()
            n201 = local write "V3"(w316) -> ()
            n202 = local write "V4"(w315) -> ()
            n203 = local write "V5"(w314) -> ()
            n204 = local write "V6"(w313) -> ()
            n205 = local write "M1-1"(w309) -> ()
            n206 = local write "M1-2"(w308) -> ()
            n207 = local write "M2"(w304) -> ()
            n208 = global write "采配水全局变量.vi" "输入状态"(w335) -> ()
            n209 = Index Array(array=w335) -> (element #1=→"X0":bool, element #2=→"X1":bool, element #3=→"X2":bool, element #4=→"X3":bool, element #5=→"X4":bool, element #6=→"X5":bool, element #7=→"X6":bool, element #8=→"X7":bool, element #9=→"X8":bool, element #10=→"X9":bool, element #11=→"X10":bool, element #12=→"X11":bool)  [unwired: 12 in]
            n210 = local write "V13NO"(w311) -> ()
            n211 = local write "V13NC"(w310) -> ()
            n212 = call <vilib>:"Read Coils.vi"("error in (no error)"=w339, "quantity"=u16 16 ("number of coils"), "starting address"=u16 2500, "MB session in"=w340) -> ("error out"=w301:errorcluster, "Coils"=w336:bool[], "MB session out"=w303:refnum<class "MB_Master.lvclass">)  [unwired: 5 in]
            n213 = global write "采配水全局变量.vi" "报警簇"(w336) -> ()
            n214 = call <vilib>:"Read Coils.vi"("error in (no error)"=w301, "quantity"=u16 1 ("starting address"), "starting address"=u16 2801, "MB session in"=w303) -> ("error out"=w300:errorcluster, "Coils"=w297:bool[], "MB session out"=w302:refnum<class "MB_Master.lvclass">)  [unwired: 5 in]
            n215 = Index Array(array=w297) -> (element=w296:bool)  [unwired: 1 in]
            n216 = local write "看门狗启用"(w296) -> ()
          }
          frame "读参数" {
            n217 = call <vilib>:"Read Holding Registers.vi"("error in (no error)"=w387, "quantity"=u16 20 ("number of holding registers"), "starting address"=u16 100, "MB session in"=w388) -> ("error out"=w382:errorcluster, "Registers"=w384:u16[], "MB session out"=w383:refnum<class "MB_Master.lvclass">)  [unwired: 5 in]
            n218 = Array To Cluster(array=w384) -> (cluster=w371:T20)
            n219 = global write "采配水全局变量.vi" "参数设置"(w371) -> ()
            n220 = Unbundle(w371) -> ("Registers[0]"=→"R100":u16, "Registers[1]"=→"R101":u16, "Registers[2]"=→"R102":u16, "Registers[3]"=→"R103":u16, "Registers[4]"=→"R104":u16, "Registers[5]"=→"R105":u16, "Registers[6]"=→"R106":u16, "Registers[7]"=→"R107":u16, "Registers[8]"=→"R108":u16, "Registers[9]"=→"R109":u16, "Registers[10]"=w370:u16, "Registers[11]"=→"R111":u16, "Registers[12]"=→"R112":u16, "Registers[13]"=→"R113":u16, "Registers[16]"=w366:u16, "Registers[18]"=→"R118":u16)  [unwired: 4 out]
            n221 = local write "R116"(w366) -> ()
            n222 = local write "潜水泵工作模式"(w370) -> ()
          }
          frame "多个写入" {
            n223 = Unbundle By Name(w394) -> ("数据"=w393:variant)
            n224 = Variant To Data(type=T14 {"starting address"=0, "holding register values"=[]}, Variant=w393) -> (data=w391:T14)  [unwired: 1 in, 1 out]
            n225 = Unbundle By Name(w391) -> ("starting address"=w390:u16, "holding register values"=w389:u16[])
            n226 = call <vilib>:"Write Multiple Registers.vi"("error in (no error)"=w397, "values"=w389, "starting address"=w390, "MB session in"=w398) -> ("error out"=w396:errorcluster, "MB session out"=w395:refnum<class "MB_Master.lvclass">)  [unwired: 6 in]
          }
          frame "单个写入" {
            n227 = Unbundle By Name(w404) -> ("数据"=w403:variant)
            n228 = Variant To Data(type=T15 {"starting address"=0, "holding register value"=0}, Variant=w403) -> (data=w401:T15)  [unwired: 1 in, 1 out]
            n229 = Unbundle By Name(w401) -> ("starting address"=w400:u16, "holding register value"=w399:u16)
            n230 = call <vilib>:"Write Single Register.vi"("error in (no error)"=w407, "value"=w399, "address"=w400, "MB session in"=w408) -> ("error out"=w406:errorcluster, "MB session out"=w405:refnum<class "MB_Master.lvclass">)  [unwired: 6 in]
          }
          frame "线圈写入" {
            n231 = Unbundle By Name(w414) -> ("数据"=w413:variant)
            n232 = Variant To Data(type=T16 {"starting address"=0, "coil values"=[]}, Variant=w413) -> (data=w411:T16)  [unwired: 1 in, 1 out]
            n233 = Unbundle By Name(w411) -> ("starting address"=w410:u16, "coil values"=w409:bool[])
            n234 = call <vilib>:"Write Multiple Coils.vi"("error in (no error)"=w417, "values"=w409, "starting address"=w410, "MB session in"=w418) -> ("error out"=w416:errorcluster, "MB session out"=w415:refnum<class "MB_Master.lvclass">)  [unwired: 6 in]
          }
          frame "shutdown" {
            n235 = call <vilib>:"Write Single Register.vi"("error in (no error)"=w428, "value"=u16 0, "address"=u16 4047, "MB session in"=w430) -> ("error out"=w429:errorcluster, "MB session out"=w427:refnum<class "MB_Master.lvclass">)  [unwired: 6 in]
            n236 = call "文件对话框"("start path"=path "D:/SRC", "pattern (all files)"="*.pdw", "pattern label"="PLC") -> ("selected path"=w424:path, "cancelled"=w422:bool)  [unwired: 9 in, 2 out]
            n237 = call-dynamic "Close Session.vi"("error in (no error)"=w429, "MB session in"=w427) -> ("error out"=w421:errorcluster)  [unwired: 9 in]
            n238 = case shown="假" w422 {
              tunnel: w424 -> [w435 _]
              tunnel: w421 -> [_ _]
              frame False {
                n239 = Path To String(path=w435) -> (string=w432:string)
                n240 = Format Into String(format string="  - \"%s\"" ("格式字符串"), initial string="\"C:\\Program Files\\Fatek\\WinProladder\\WProlad.exe\"" ("command line"), w432) -> (resulting string=w433:string)  [unwired: 1 in, 1 out]
                n241 = call <vilib>:"System Exec.vi"("command line"=w433) -> ("error out"=w436:errorcluster)  [unwired: 7 in, 3 out]
                n242 = case shown="错误" w436 {
                  tunnel: w432 -> [_ w439]
                  frame No Error {
                  }
                  frame Error {
                    n243 = Format Into String(format string="  - \"%s\"" ("格式字符串"), initial string="\"C:\\Program Files (x86)\\Fatek\\WinProladder\\WProlad.exe\"" ("command line"), w439) -> (resulting string=w437:string)  [unwired: 1 in, 1 out]
                    n244 = call <vilib>:"System Exec.vi"("command line"=w437) -> ()  [unwired: 7 in, 4 out]
                  }
                }
              }
              frame True {
              }
            }
          }
        }
      }
      frame Error {
        n245 = Unbundle By Name(w445) -> ("code"=w447:i32)
        n246 = case shown="-1073807343" w447 {
          tunnel: w446 -> [w449 w453]
          tunnel: w445 -> [w448 w455]
          tunnel: [w448 w454] -> w443
          tunnel: [w449 w453] -> w444
          tunnel: w441 -> [_ w452]
          frame Default {
          }
          frame -1073807343 {
            n247 = Flush Queue(queue=w452) -> (queue out=w451:refnum<queue>)  [unwired: 1 in, 2 out]
            n248 = call-dynamic "Close Session.vi"("error in (no error)"=w455, "MB session in"=w453) -> ("error out"=w454:errorcluster)  [unwired: 9 in]
            n249 = disable-structure shown="禁用" {
              disable-tunnel: w451 -> [w456 _]
              frame Disabled {
                n250 = Enqueue Element At Opposite End(queue=w456, element=cluster{"命令":string, "数据":variant} {"命令"="init", "数据"=variant} ("元素")) -> ()  [unwired: 2 in, 3 out]
              }
              frame Enabled {
              }
            }
            n251 = Wait (ms)(milliseconds to wait=u32 2000 ("等待时间（毫秒）")) -> ()  [unwired: 1 out]
          }
        }
        n252 = call <vilib>:"Clear Errors.vi"("error in (no error)"=w443) -> ("error out"=w442:errorcluster)  [unwired: 5 in, 1 out]
      }
    }
    n253 = Unbundle By Name(w251) -> ("status"=→"通讯故障":bool)
  }
  n254 = property on="多列列表框" class="MCListbox (严格)"("ItemNames"=string[][] [["待机"], ["初始化"], ["外部管路润洗"], ["内部管路润洗"], ["采样"], ["沉淀"], ["配水"], ["外部管路反冲洗"], ["内部管路反冲洗"], ["采样池储水"], ["结束"]] ("项名")) -> ()  [unwired: 2 in, 2 out]
  n255 = while {
    shift-right: [w463] -> _
    shift-left: _ -> [w465]
    shift-right: [w462] -> _
    shift-left: _ -> [w464]
    shift-right: [w459] -> _
    shift-left: enum16{"open", "read", "write", "close"}."open" -> [w460]
    stop <- FALSE stop-if-true
    # "模块为主站modbustcp地址与其他模块交互\n1氨氮  2总磷 3总氮 4CODMn 5CODCr 10采配水"
    n256 = Wait (ms)(milliseconds to wait=u32 1000 ("等待时间（毫秒）")) -> ()  [unwired: 1 out]
    n257 = case shown="\"open\", 默认" w460 {
      selector: w460 -> [w474 _ _ _]
      tunnel: w465 -> [w468 w480 w491 w497]
      tunnel: w464 -> [w467 w479 w488 w496]
      tunnel: [w471 w477 w487 w497] -> w463
      tunnel: [w470 w478 w486 w499] -> w462
      tunnel: [w473 w483 w492 enum16{"open", "read", "write", "close"}."open"] -> w459
      frame "open", Default {
        n258 = call-dynamic "Shutdown.vi"("error in"=w467, "Modbus slave in"=w468) -> ("error out"=w466:errorcluster)  [unwired: 9 in]
        n259 = call <vilib>:"Clear Errors.vi"("error in (no error)"=w466) -> ("error out"=w469:errorcluster)  [unwired: 5 in, 1 out]
        n260 = call-poly <vilib>:"Create Modbus Instance.vi"("error in"=w469, "port (502)"=u16 10) -> ("error out"=w470:errorcluster, "TCP slave instance"=w471:refnum<class "Modbus Slave.lvclass">)  [unwired: 8 in]
        n261 = case shown="无错误" w470 {
          tunnel: w474 -> [_ w476]
          tunnel: [enum16{"open", "read", "write", "close"}."write" w476] -> w473
          frame No Error {
          }
          frame Error {
          }
        }
      }
      frame "read" {
        n262 = call-dynamic <vilib>:"Read Holding Registers.vi"("error in"=w479, "number of inputs"=u16 1, "starting address"=u16 257, "Modbus slave in"=w480) -> ("error out"=w478:errorcluster, "Modbus slave out"=w477:refnum<class "Modbus Slave.lvclass">)  [unwired: 5 in, 1 out]
        n263 = case shown="无错误" w478 {
          tunnel: [enum16{"open", "read", "write", "close"}."write" enum16{"open", "read", "write", "close"}."close"] -> w483
          frame No Error {
          }
          frame Error {
          }
        }
      }
      frame "write" {
        n264 = local read "Registers"() -> (w489:u16[])
        n265 = call-dynamic "Write Multiple Holding Registers.vi"("error in"=w488, "registers to write"=w489, "starting address"=u16 0, "Modbus slave in"=w491) -> ("error out"=w486:errorcluster, "Modbus slave out"=w487:refnum<class "Modbus Slave.lvclass">)  [unwired: 6 in]
        n266 = case shown="无错误" w486 {
          tunnel: [enum16{"open", "read", "write", "close"}."write" enum16{"open", "read", "write", "close"}."close"] -> w492
          frame No Error {
          }
          frame Error {
          }
        }
      }
      frame "close" {
        n267 = call-dynamic "Shutdown.vi"("error in"=w496, "Modbus slave in"=w497) -> ("error out"=w495:errorcluster)  [unwired: 9 in]
        n268 = call <vilib>:"Clear Errors.vi"("error in (no error)"=w495) -> ("error out"=w499:errorcluster)  [unwired: 5 in, 1 out]
      }
    }
  }
  n269 = call-dynamic "Close Session.vi"("error in (no error)"=w6, "MB session in"=w5) -> ()  [unwired: 9 in, 1 out]
